vi "Fmt_ExitWithCode.vi"(8 "error in (no error)":errorcluster) -> (3 "<JSON>":string)   [LabVIEW 2020]
uses:
  8fd20af5-7dae-4bf1-85d1-60bdefd233dc.vi
  <vilib>/JDP Science/JSONtext/Variant to JSON Text.vi
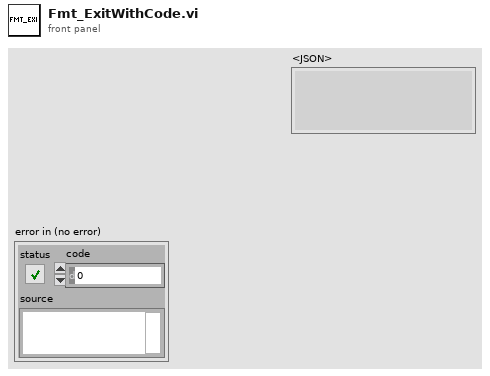
[diagram p1: front panel]
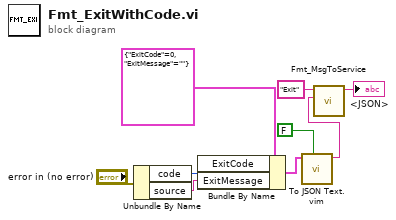
[diagram p0: block diagram]
diagram:
  n1 = Unbundle By Name("error in (no error)") -> ("code"=w4:i32, "source"=w2:string)
  n2 = Bundle By Name(cluster=cluster{"ExitCode":i32, "ExitMessage":string} {"ExitCode"=0, "ExitMessage"=""}, "ExitCode"=w4, "ExitMessage"=w2) -> (w7:cluster{"ExitCode":i32, "ExitMessage":string})
  n3 = call "To JSON Text.vim"("enable LabVIEW extensions? (T)"=FALSE, "Anything"=w7) -> ("<JSON>"=w6:string)  [unwired: 8 in, 1 out]
  n4 = call "Fmt_MsgToService.vi"("Data"=w6, "state"="Exit") -> ("<JSON>"=→"<JSON>":string)  [unwired: 9 in]
